vi "FormatCommand.vi"(11 "Command":string) -> (2 "CRC":u16 format="%.0x", 3 "Formatted Command":string)   [LabVIEW 2012, in "Sierra-M100.lvlib"]
doc: "This VI properly formats an ASCII command with the command, the value, the CRC, and a carriage return."
uses:
  Sierra-M100.lvlib
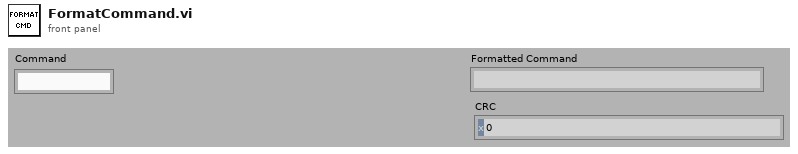
[diagram p1: front panel]
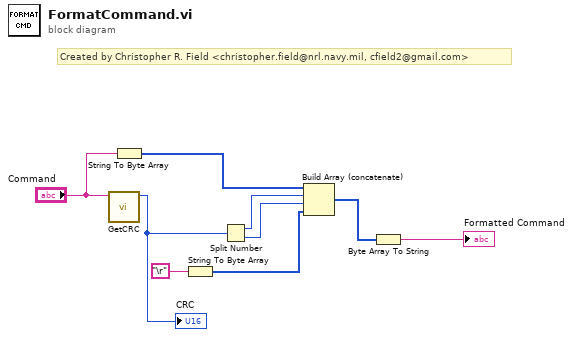
[diagram p0: block diagram]
diagram:
  # "Created by Christopher R. Field <christopher.field@nrl.navy.mil, cfield2@gmail.com>"
  n1 = call "GetCRC.vi"("Command"="Command") -> ("CRC"=w7:u16)  [unwired: 10 in]
  "CRC" <- w7
  n2 = String To Byte Array(string="Command") -> (unsigned byte array=w8:u8[])
  n3 = String To Byte Array(string="\r") -> (unsigned byte array=w3:u8[])
  n4 = Split Number(x=w7) -> (hi(x)=w6:u8, lo(x)=w5:u8)
  n5 = Build Array (concatenate)(w8, w6, w5, w3) -> (w2:u8[])
  n6 = Byte Array To String(unsigned byte array=w2) -> (string=→"Formatted Command":string)
